vi "IntakeForTimeController.vi"(6 "Start Time (ms)":u32, 9 "Current TIme":u32, 10 "Speed in":dbl, 11 "Duration":dbl) -> (1 "Delay":dbl, 2 "Done":bool, 3 "Speed out":dbl)   [LabVIEW 2018]
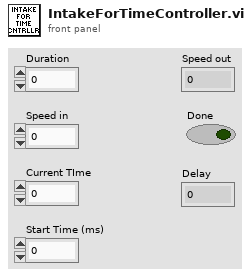
[diagram p1: front panel]
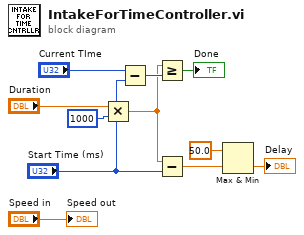
[diagram p0: block diagram]
diagram:
  n1 = Multiply(x="Duration", y=1000) -> (x*y=w3:dbl)
  n2 = Subtract(x="Current TIme", y="Start Time (ms)") -> (x-y=w4:u32)
  n3 = Greater Or Equal?(x=w3, y=w4) -> (x >= y?=→"Done":bool)
  n4 = Subtract(x=w3, y="Start Time (ms)") -> (x-y=w1:dbl)
  n5 = Max & Min(x=50.0, y=w1) -> (min(x,y)=→"Delay":dbl)  [unwired: 1 out]
  "Speed out" <- "Speed in"
